vi "XmlRpcRequestCallbackVI.vi"(4 "Answer number":refnum<vi>, 5 "Event Data":T1, 6 "Control Ref":refnum<k24>, 7 "Event Common Data":T2) -> ()   [LabVIEW 2016]
uses:
  C:/Users/fg/Documents/UniversalRobots.vi/LabVIEW_2024/UnderAutomation.UniversalRobots/lib/UnderAutomation.UniversalRobots.dll
  LabVIEW_2024/UnderAutomation.UniversalRobots/lib/UnderAutomation.UniversalRobots.dll
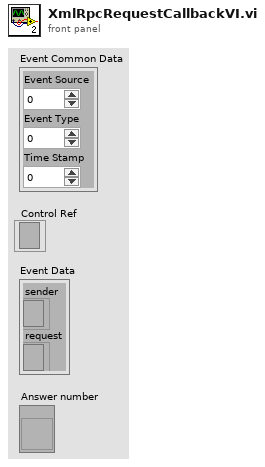
[diagram p1: front panel]
types:
  T1 = cluster{"sender":refnum<k24>, "request":refnum<k24>}
  T2 = cluster{"Event Source":i32, "Event Type":u32, "Time Stamp":u32}
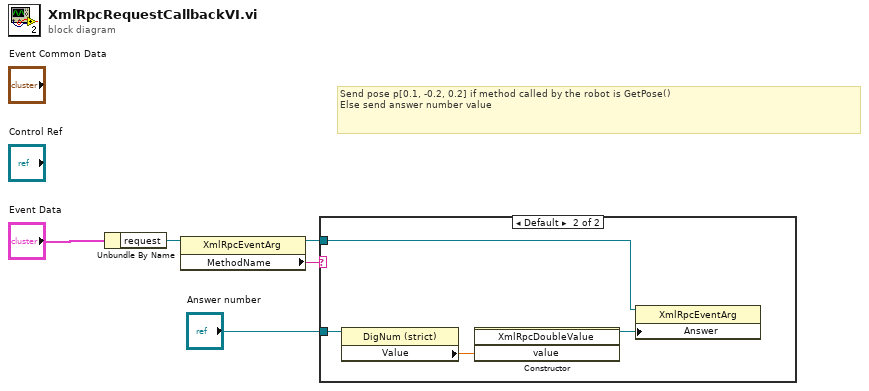
[diagram p0: block diagram]
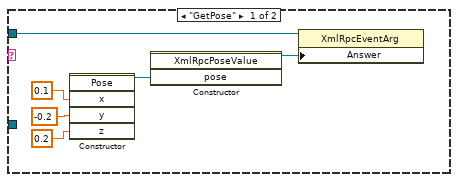
[diagram p2: hidden frame]
diagram:
  # "Send pose p[0.1, -0.2, 0.2] if method called by the robot is GetPose()\nElse send answer number value"
  n1 = Unbundle By Name("Event Data") -> ("request"=w4:refnum<k24>)
  n2 = property class="XmlRpcEventArg"(reference=w4) -> (reference out=w1:refnum<k24>, "MethodName"=w3:string)  [unwired: 1 in, 1 out]
  n3 = case shown="Default" w3 {
    tunnel: "Answer number" -> [_ w15]
    tunnel: w1 -> [w7 w12]
    frame "GetPose" {
      n4 = constructor class="Pose"("x"=0.1, "y"=-0.2, "z"=0.2) -> (reference out=w8:refnum<k24>)  [unwired: 3 in, 5 out]
      n5 = constructor class="XmlRpcPoseValue"("pose"=w8) -> (reference out=w6:refnum<k24>)  [unwired: 3 in, 3 out]
      n6 = property class="XmlRpcEventArg"(reference=w7, "Answer"=w6) -> ()  [unwired: 1 in, 2 out]
    }
    frame Default {
      n7 = property class="DigNum (strict)"(reference=w15) -> ("Value"=w14:dbl)  [unwired: 1 in, 2 out]
      n8 = constructor class="XmlRpcDoubleValue"("value"=w14) -> (reference out=w13:refnum<k24>)  [unwired: 3 in, 3 out]
      n9 = property class="XmlRpcEventArg"(reference=w12, "Answer"=w13) -> ()  [unwired: 1 in, 2 out]
    }
  }
